vi "dvp Vi Set Stream State.vi"(10 "StreamState":u32(ring) items=["STATE_STOPED", "STATE_PAUSED", "STATE_STARTED"], 11 "handle":u32) -> (3 "function return":u32(ring))   [LabVIEW 2018, in "LabViewDVPCamera.lvlib"]
doc: "LabviewDvp2Api dvpStatus dvpViSetStreamState(dvpHandle handle, dvpStreamState StreamState);"
uses:
  LabViewDVPCamera.lvlib
  LabViewDVPCamera/LabViewDVPCamera.dll
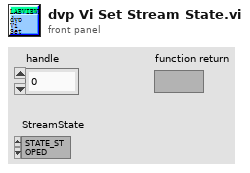
[diagram p1: front panel]
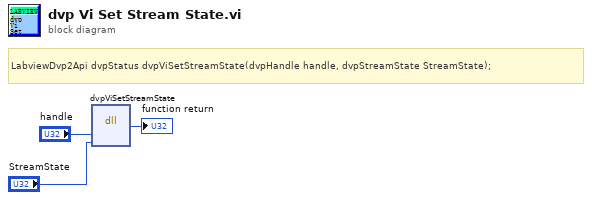
[diagram p0: block diagram]
diagram:
  # "LabviewDvp2Api dvpStatus dvpViSetStreamState(dvpHandle handle, dvpStreamState StreamState);"
  n1 = dll-call lib="C:/Program Files (x86)/DVP2 Labview cn 64/Sample/LabViewDVPCamera/LabViewDVPCamera.*" fn="dvpViSetStreamState"("handle"="handle", "StreamState"="StreamState") -> (→"function return":u32)  [unwired: 5 in, 2 out]
